vi "test_alignHorizontalCentersValidation.vi"(11 "Test Case In":refnum<class "AlignmentTests.lvclass">) -> (0 "error out":errorcluster, 3 "Test Case Out":refnum<class "AlignmentTests.lvclass">)   [LabVIEW 2023, in "AlignmentTests.lvclass"]
uses:
  AlignmentTests.lvclass
  <vilib>/Astemes/LUnit/Test Case.lvclass/Test Case.ctl
  <vilib>/Astemes/LUnit/Core/LUnit Test Case/Private/Append Fail Result.vi
  <vilib>/Astemes/LUnit/Core/LUnit Test Case/Private/Append Pass Result.vi
  <vilib>/Astemes/LUnit/Core/LUnit Test Case/Private/Run In UI.vi
  <vilib>/Utility/error.llb/Clear Errors.vi
  AlignmentTests.lvclass/AlignmentTests.ctl
  <vilib>/Astemes/LUnit/Test Case.lvclass
panel:
  in  "Numeric 3":dbl
  in  "Numeric 2":dbl
  in  "Numeric":dbl
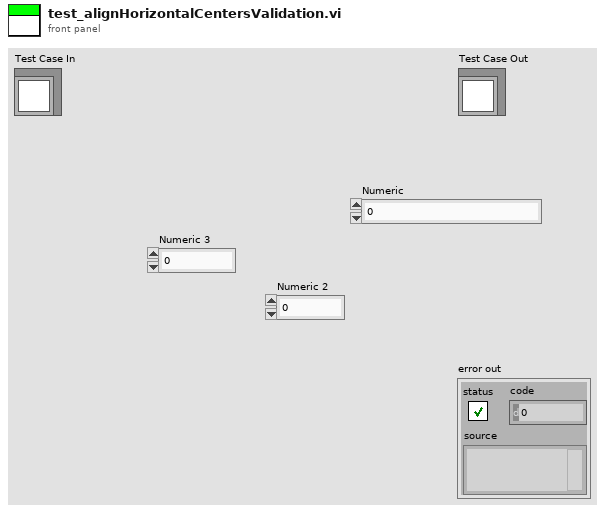
[diagram p1: front panel]
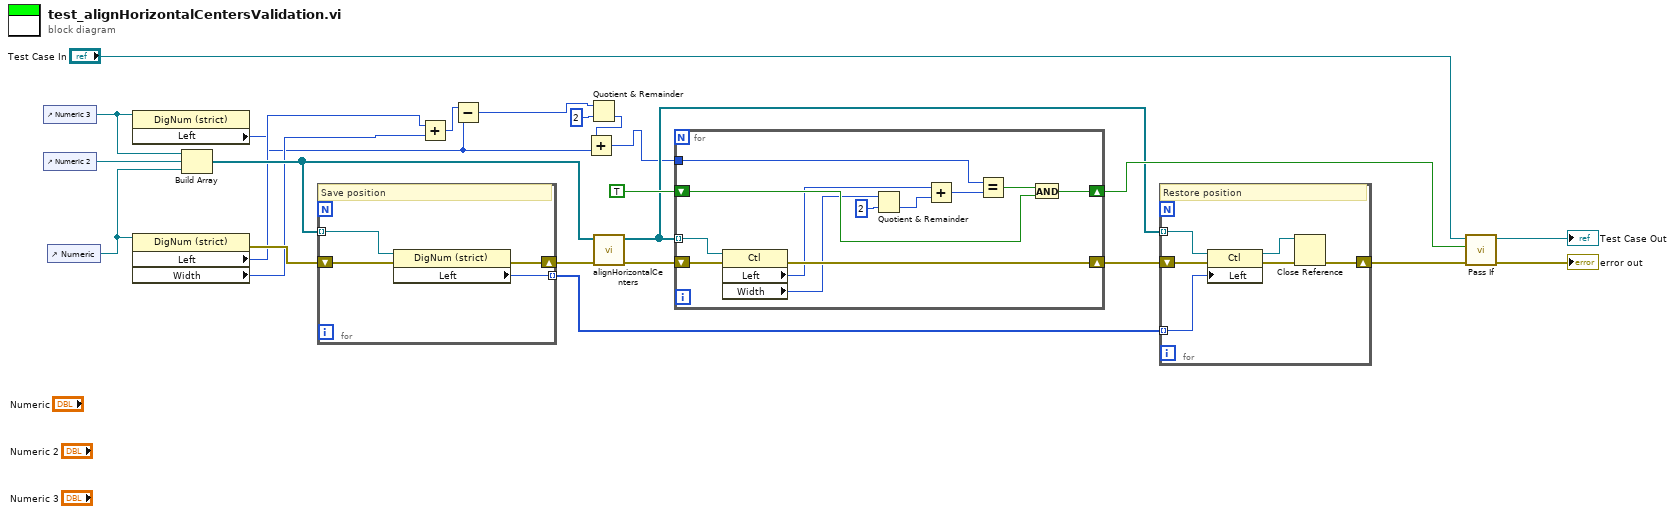
[diagram p0: block diagram]
diagram:
  n1 = control-ref of="Numeric 3"() -> (w10:refnum<vi>)
  n2 = control-ref of="Numeric 2"() -> (w21:refnum<vi>)
  n3 = control-ref of="Numeric"() -> (w9:refnum<vi>)
  n4 = property class="DigNum (strict)"(reference=w10) -> ("Left"=w1:i32)  [unwired: 1 in, 2 out]
  n5 = property class="DigNum (strict)"(reference=w9) -> (error out=w17:errorcluster, "Left"=w8:i32, "Width"=w7:u32)  [unwired: 1 in, 1 out]
  n6 = Build Array(w10, w21, w9) -> (w12:refnum<vi>[])
  n7 = for {
    tunnel: w12 -> [w28] mode=indexing
    shift-right: [w26] -> w16
    shift-left: w17 -> [w27]
    tunnel: [w25] -> w13 mode=indexing
    # "Save position"
    n8 = property class="DigNum (strict)"(reference=w28, error in=w27) -> (error out=w26:errorcluster, "Left"=w25:i32)  [unwired: 1 out]
  }
  n9 = Add(x=w8, y=w7) -> (x+y=w3:u32)
  n10 = Subtract(x=w3, y=w1) -> (x-y=w5:u32)
  n11 = Quotient & Remainder(x=w5, y=u32 2) -> (floor(x/y)=w4:u32)  [unwired: 1 out]
  n12 = Add(x=w4, y=w1) -> (x+y=w2:u32)
  n13 = call "alignHorizontalCenters.vi"("error in (no error)"=w16, "refs"=w12) -> ("error out"=w18:errorcluster, "refs(dup)"=w11:refnum<vi>[])  [unwired: 8 in]
  n14 = for {
    tunnel: w11 -> [w40] mode=indexing
    tunnel: w2 -> [w39]
    shift-right: [w37] -> w19
    shift-left: TRUE -> [w36]
    shift-right: [w34] -> w14
    shift-left: w18 -> [w35]
    n15 = property class="Ctl"(reference=w40, error in=w35) -> (error out=w34:errorcluster, "Left"=w33:i32, "Width"=w30:u32)  [unwired: 1 out]
    n16 = Quotient & Remainder(x=w30, y=u32 2) -> (floor(x/y)=w29:u32)  [unwired: 1 out]
    n17 = Add(x=w33, y=w29) -> (x+y=w32:u32)
    n18 = Equal?(x=w39, y=w32) -> (x = y?=w38:bool)
    n19 = And(x=w38, y=w36) -> (x .and. y?=w37:bool)
  }
  n20 = for {
    tunnel: w11 -> [w46] mode=indexing
    shift-right: [w42] -> w15
    shift-left: w14 -> [w45]
    tunnel: w13 -> [w43] mode=indexing
    # "Restore position"
    n21 = property class="Ctl"(reference=w46, error in=w45, "Left"=w43) -> (reference out=w41:refnum<vi>, error out=w44:errorcluster)
    n22 = Close Reference(reference=w41, error in (no error)=w44) -> (error out=w42:errorcluster)
  }
  n23 = call <vilib>:"Pass If.vi"("error in (no error)"=w15, "Pass?"=w19, "LUnit Test Case In"="Test Case In") -> ("error out"=→"error out":errorcluster, "LUnit Test Case Out"=→"Test Case Out":refnum<class "AlignmentTests.lvclass">)  [unwired: 7 in]
